vi "Write Conversion Log File.vi"(5 "End time":timestamp, 6 "Additional Notes?":string, 7 "Start time":timestamp, 8 "error in (no error)":errorcluster, 9 "Failed Converted Files":path[](array[path]), 10 "Converted Files":path[](array[path]), 11 "Original Files":path[](array[path])) -> (0 "error out":errorcluster, 3 "Log File Path":path)   [LabVIEW 2016]
uses:
  <userlib>/_OpenG.lib/file/file.llb/Strip Path - Arrays__ogtk.vi
  <userlib>/_OpenG.lib/array/array.llb/Remove Duplicates from 1D Array (Path)__ogtk.vi
panel:
  out "resulting string":string
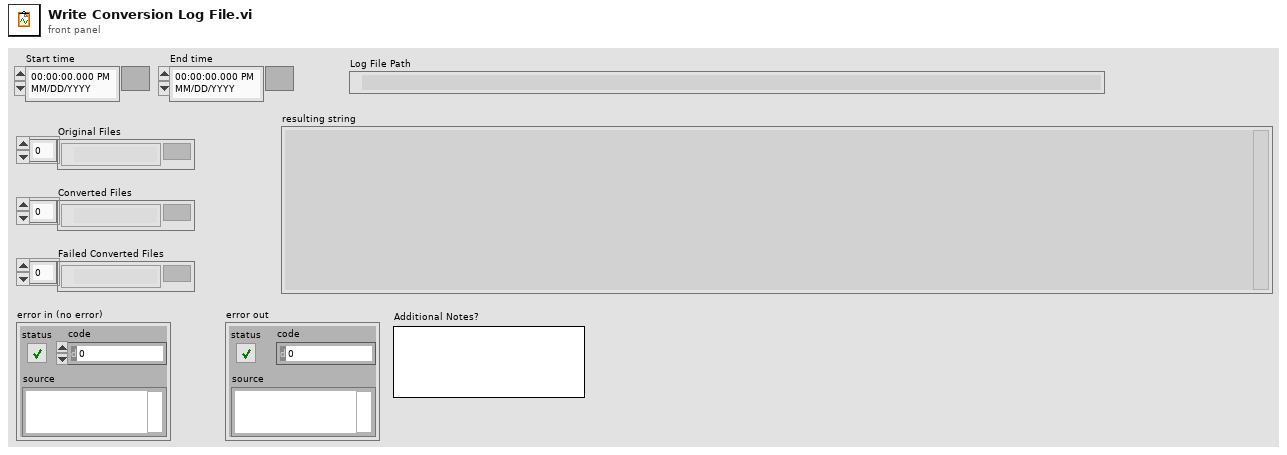
[diagram p1: front panel]
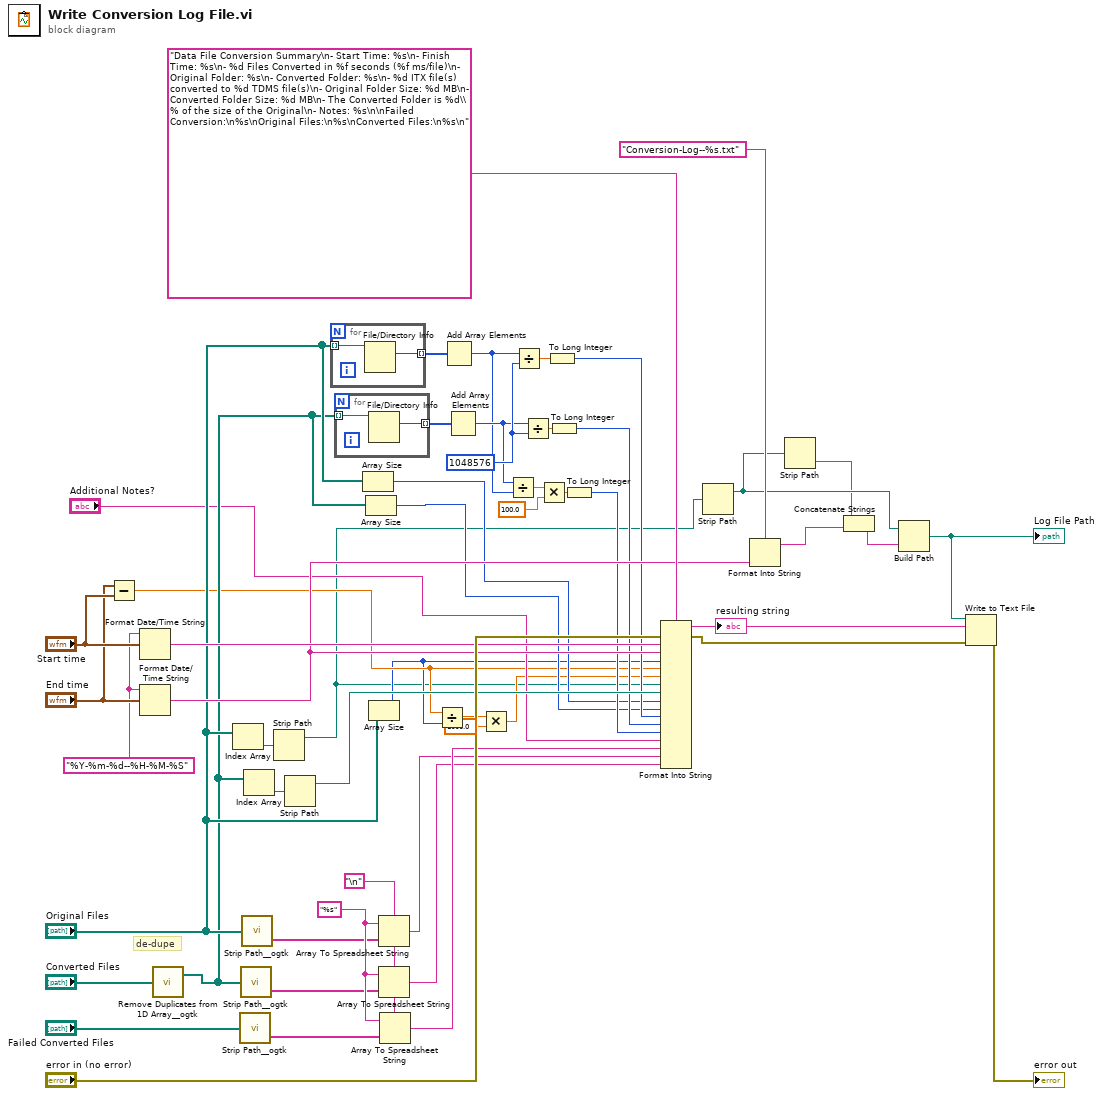
[diagram p0: block diagram]
diagram:
  w30 = i64 1048576 ("y")
  w35 = "%Y-%m-%d--%H-%M-%S" ("time format string (%c)")
  w50 = "%s" ("format string")
  w53 = "\n"
  # "de-dupe"
  n1 = Subtract(x="End time", y="Start time") -> (x-y=w10:dbl)
  n2 = Format Date/Time String(time format string (%c)=w35, seconds (now)="Start time") -> (date/time string=w37:string)  [unwired: 1 in]
  n3 = Format Date/Time String(time format string (%c)=w35, seconds (now)="End time") -> (date/time string=w36:string)  [unwired: 1 in]
  n4 = call-poly <userlib>:"Remove Duplicates from 1D Array__ogtk.vi"("Input Array"="Converted Files") -> ("Output Array"=w13:path[])  [unwired: 1 out]
  n5 = Index Array(array="Original Files") -> (element=w49:path)  [unwired: 1 in]
  n6 = call-poly <userlib>:"Strip Path__ogtk.vi"("path"="Failed Converted Files") -> ("name"=w45:string[])  [unwired: 1 out]
  n7 = call-poly <userlib>:"Strip Path__ogtk.vi"("path"=w13) -> ("name"=w46:string[])  [unwired: 1 out]
  n8 = call-poly <userlib>:"Strip Path__ogtk.vi"("path"="Original Files") -> ("name"=w48:string[])  [unwired: 1 out]
  n9 = Index Array(array=w13) -> (element=w41:path)  [unwired: 1 in]
  n10 = Strip Path(path=w49) -> (stripped path=w5:path)  [unwired: 1 out]
  n11 = Strip Path(path=w41) -> (stripped path=w33:path)  [unwired: 1 out]
  n12 = for {
    tunnel: [w55] -> w34 mode=indexing
    tunnel: "Original Files" -> [w54] mode=indexing
    n13 = File/Directory Info(path=w54) -> (size=w55:i64)  [unwired: 1 in, 6 out]
  }
  n14 = for {
    tunnel: [w57] -> w32 mode=indexing
    tunnel: w13 -> [w56] mode=indexing
    n15 = File/Directory Info(path=w56) -> (size=w57:i64)  [unwired: 1 in, 6 out]
  }
  n16 = Array Size(array="Original Files") -> (size(s)=w14:i32)
  n17 = Array Size(array=w13) -> (size(s)=w12:i32)
  n18 = Array Size(array="Original Files") -> (size(s)=w9:i32)
  n19 = Array To Spreadsheet String(delimiter (Tab)=w53, array=w48, 3:w50) -> (spreadsheet string=w43:string)
  n20 = Array To Spreadsheet String(delimiter (Tab)=w53, array=w46, 3:w50) -> (spreadsheet string=w42:string)
  n21 = Array To Spreadsheet String(delimiter (Tab)=w53, array=w45, 3:w50) -> (spreadsheet string=w44:string)
  n22 = Divide(x=w10, y=w9) -> (x/y=w8:dbl)
  n23 = Add Array Elements(numeric array=w34) -> (sum=w25:i64)
  n24 = Add Array Elements(numeric array=w32) -> (sum=w26:i64)
  n25 = Multiply(x=w8, y=1000.0) -> (x*y=w6:dbl)
  n26 = Divide(x=w26, y=w25) -> (x/y=w24:dbl)
  n27 = Divide(x=w25, y=w30) -> (x/y=w31:dbl)
  n28 = Divide(x=w26, y=w30) -> (x/y=w29:dbl)
  n29 = Multiply(x=w24, y=100.0) -> (x*y=w22:dbl)
  n30 = To Long Integer(number=w31) -> (32bit integer=w28:i32)
  n31 = To Long Integer(number=w29) -> (32bit integer=w27:i32)
  n32 = To Long Integer(number=w22) -> (32bit integer=w21:i32)
  n33 = Format Into String(format string="Data File Conversion Summary\n- Start Time: %s\n- Finish Time: %s\n- %d Files Converted in %f seconds (%f ms/file)\n- Original Folder: %s\n- Converted Folder: %s\n- %d ITX file(s) converted to %d TDMS file(s)\n- Original Folder Size: %d MB\n- Converted Folder Size: %d MB\n- The Converted Folder is %d\\% of the size of the Original\n- Notes: %s\n\nFailed Conversion:\n%s\nOriginal Files:\n%s\nConverted Files:\n%s\n", error in="error in (no error)", w37, w36, w9, w10, w6, w5, w33, w14, w12, w28, w27, w21, "Additional Notes?", w44, w43, w42) -> (resulting string=w17:string, error out=w20:errorcluster)  [unwired: 1 in]
  "resulting string" <- w17
  n34 = Strip Path(path=w5) -> (stripped path=w4:path)  [unwired: 1 out]
  n35 = Format Into String(format string="Conversion-Log--%s.txt" ("name or relative path"), w36) -> (resulting string=w2:string)  [unwired: 2 in, 1 out]
  n36 = Strip Path(path=w4) -> (name=w3:string)  [unwired: 1 out]
  n37 = Concatenate Strings(w3, w2) -> (w1:string)
  n38 = Build Path(base path=w4, name or relative path=w1) -> (appended path=w18:path)
  "Log File Path" <- w18
  n39 = Write to Text File(file (use dialog)=w18, text=w17, error in=w20) -> (error out=→"error out":errorcluster)  [unwired: 1 in, 2 out]
